vi "Window Picker.vi"() -> (2 "Selected?":bool, 3 "Selection":T1[](array[typedef]) {"Plot Bounds (%)"."Bottom (%)" format="%.2f"; "Plot Bounds (%)"."Top (%)" format="%.2f"; "Plot Bounds (%)"."Right (%)" format="%.2f"; "Plot Bounds (%)"."Left (%)" format="%.2f"})   [LabVIEW 2021, in "MultiRocketPlotPanel.lvclass"]
uses:
  Classes/MultiPlotPanel/MultiRocketPlotPanel.lvclass
  Window Position and plot number.ctl
  Window Position.ctl
  <vilib>/Utility/miscctls.llb/LVRowAndColumnTypeDef.ctl
  Panel Movement Center Maximize/Panel Movement Center Maximize.lvlib
panel:
  out "Options":picture[][](array[picture])
  in  "Select (spoof)":bool
  in  "Select":bool
  in  "Cancel":bool
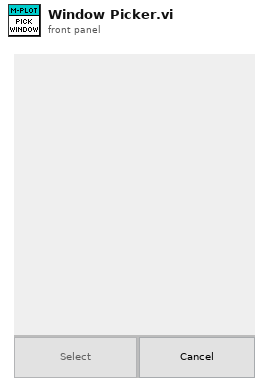
[diagram p1: front panel]
types:
  T1 = typedef "MultiRocketPlotPanel.lvclass/Window Position and plot number.ctl" = cluster{"Plot Number":i32, "Plot Bounds (%)":T2}
  T2 = typedef "MultiRocketPlotPanel.lvclass/Window Position.ctl" = cluster{"Left (%)":dbl, "Top (%)":dbl, "Right (%)":dbl, "Bottom (%)":dbl}
  T3 = typedef "LVRowAndColumnTypeDef.ctl" = cluster{"Row":i32, "Column":i32}
  T4 = enum8{"Enabled", "Disabled", "Disabled and Grayed Out"}
  T5 = typedef "LVPoint32TypeDef.ctl" = cluster{"Horizontal":i32, "Vertical":i32}
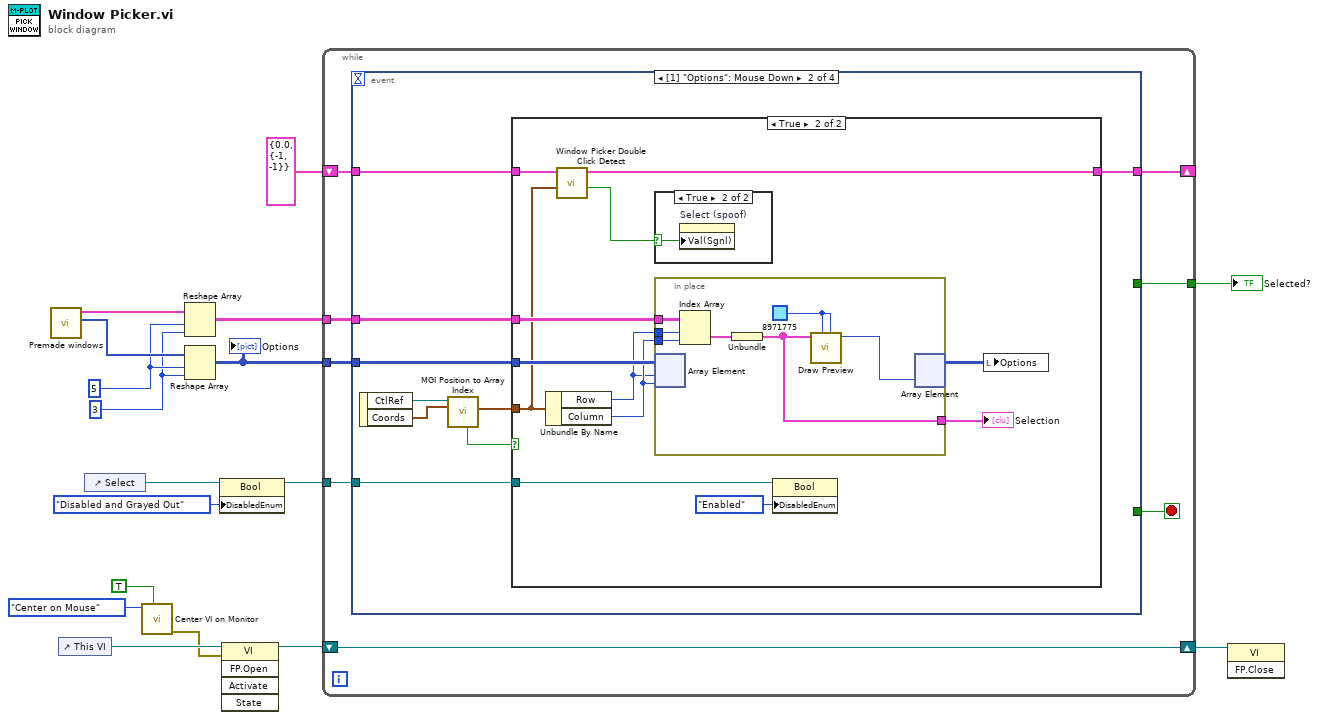
[diagram p0: block diagram]
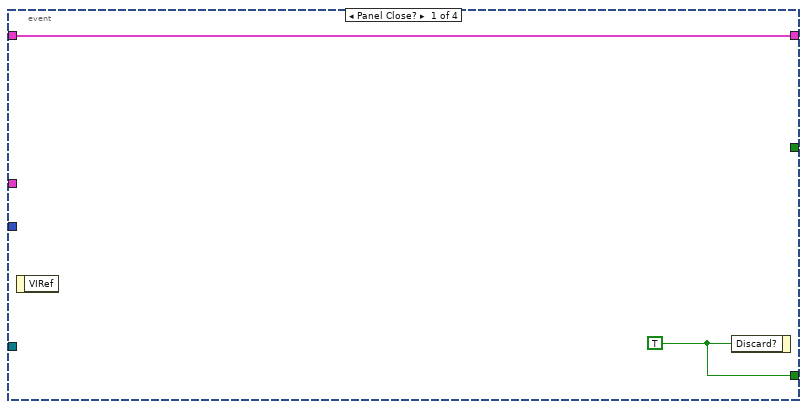
[diagram p2: hidden frame]
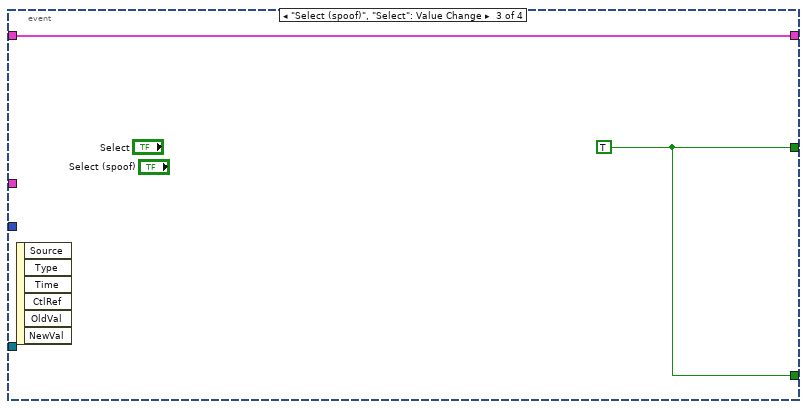
[diagram p5: hidden frame]
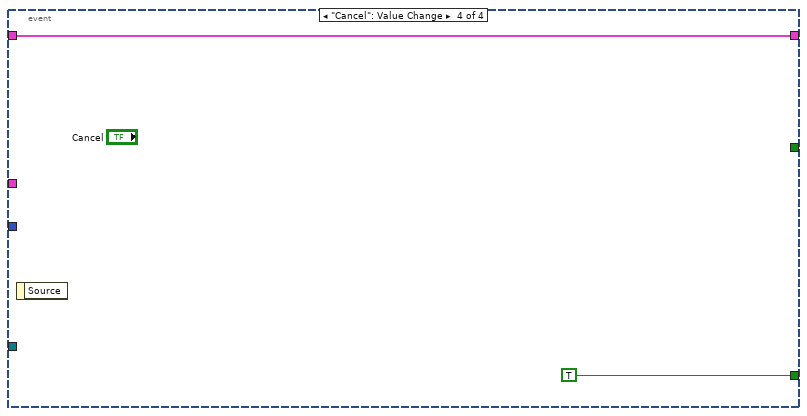
[diagram p6: hidden frame]
diagram:
  w5 = 5 ("dimension size")
  w4 = 3 ("dimension size")
  n1 = call "Premade windows.vi"() -> ("Premade Windows (pic)"=w17:picture[], "Premade Windows"=w15:cluster{"Plot Bounds":T1[]}[])  [unwired: 10 in]
  n2 = control-ref of="This VI"() -> (w7:refnum<vi>)
  n3 = control-ref of="Select"() -> (w13:refnum<vi>)
  n4 = call "Center VI on Monitor.vi"("Make Modal"=TRUE, "Window Mode (Center on Monitor)"=enum16{"Center on Monitor", "Center on Mouse"}."Center on Mouse") -> ("error out"=w1:errorcluster)  [unwired: 9 in]
  n5 = Reshape Array(w15, w5, w4) -> (w14:cluster{"Plot Bounds":T1[]}[][])
  n6 = Reshape Array(w17, w5, w4) -> (w16:picture[][])
  "Options" <- w16
  n7 = property class="Bool"(reference=w13, "DisabledEnum"=T4."Disabled and Grayed Out" ("Disabled")) -> (reference out=w9:refnum<vi>)  [unwired: 1 in, 1 out]
  n8 = invoke class="VI" method="FP.Open"(reference=w7, error in=w1) -> (reference out=w6:refnum<vi>)  [unwired: 3 in, 4 out]
  n9 = while {
    tunnel: w16 -> [w24]
    tunnel: w14 -> [w23]
    shift-right: [w22] -> w11
    shift-left: w6 -> [w22]
    tunnel: [w21] -> w10
    tunnel: w9 -> [w20]
    shift-right: [w18] -> _
    shift-left: cluster{dbl, "Index":T3} {0.0, "Index"={"Row"=-1, "Column"=-1}} -> [w19]
    stop <- w25 stop-if-true
    n10 = event shown="[1] \"Options\": Mouse Down" {
      selector: _ -> [_ _ _ _]
      dyn-events: _ -> [_ _ _ _]
      timeout: _ -> [_ _ _ _]
      tunnel: [w27 _ w59 TRUE ("Discard?")] -> w25
      tunnel: w24 -> [_ w34 _ _]
      tunnel: w23 -> [_ w32 _ _]
      tunnel: [_ _ w59 _] -> w21
      tunnel: w20 -> [_ w31 _ _]
      tunnel: w19 -> [w26 w29 w58 w60]
      tunnel: [w26 w28 w58 w60] -> w18
      event Panel Close? {
        w27 = TRUE ("Discard?")
        n11 = event-data() -> ()  [unwired: 1 in, 1 out]
        n12 = event-data("Discard?"=w27) -> ()  [unwired: 1 in, 1 out]
      }
      event "Options": Mouse Down {
        n13 = event-data() -> ("CtlRef"=w36:refnum<vi>, "Coords"=w35:T5)  [unwired: 1 in]
        n14 = call <userlib>:"MGI Position to Array Index.vi"("Coords"=w35, "ArrayRef"=w36) -> ("Index"=w33:T3, "In Bounds?"=w30:bool)  [unwired: 5 in, 3 out]
        n15 = case shown="True" w30 {
          tunnel: w34 -> [_ w49]
          tunnel: w33 -> [_ w40]
          tunnel: w32 -> [_ w48]
          tunnel: w31 -> [_ w43]
          tunnel: w29 -> [w37 w41]
          tunnel: [w37 w39] -> w28
          frame False {
          }
          frame True {
            n16 = Unbundle By Name(w40) -> ("Row"=w46:i32, "Column"=w47:i32)
            n17 = call "Window Picker Double Click Detect.vi"("Index (mouse down)"=w40, "Loop data (previous)"=w41) -> ("Double Clicked?"=w38:bool, "Loop data (new)"=w39:cluster{"timestamp":dbl, "Index":T3})  [unwired: 8 in]
            n18 = case shown="True" w38 {
              selector: w38 -> [_ w50]
              frame False {
              }
              frame True {
                n19 = property on="Select (spoof)" class="Bool (strict)"("Val(Sgnl)"=w50) -> ()  [unwired: 2 in, 2 out]
              }
            }
            n20 = in-place {
              in-place-border: w48 -> [w57]
              in-place-border: w47 -> [w56]
              in-place-border: w46 -> [w55]
              in-place-border: [w51] -> w44
              w52 = u32 8971775
              n21 = in-place-array #1(w49, w46, w47) -> ()  [unwired: 1 out]
              n22 = Index Array(array=w57, index (row)=w55, index (col)=w56) -> (element=w54:cluster{"Plot Bounds":T1[]})
              n23 = Unbundle(w54) -> ("Plot Bounds"=w51:T1[])
              n24 = call "Draw Preview.vi"("BG Color"=w52, "Box Color"=w52, "Plot Bounds"=w51) -> ("Preview Pict"=w53:picture)  [unwired: 8 in]
              n25 = in-place-array #1(w53) -> (w45:picture[][])  [unwired: 2 out]
            }
            "Selection" <- w44
            n26 = property class="Bool"(reference=w43, "DisabledEnum"=T4."Enabled" ("Disabled")) -> ()  [unwired: 1 in, 2 out]
            n27 = local write "Options"(w45) -> ()
          }
        }
      }
      event "Select (spoof)", "Select": Value Change {
        w59 = TRUE
        n28 = event-data() -> ()  [unwired: 1 in, 6 out]
      }
      event "Cancel": Value Change {
        n29 = event-data() -> ()  [unwired: 1 in, 1 out]
      }
    }
  }
  "Selected?" <- w10
  n30 = invoke class="VI" method="FP.Close"(reference=w11) -> ()  [unwired: 2 in, 3 out]
